vi "Search for Target.vi"(0 "Target":T2, 1 "Focus and Tracking":T3, 3 "Calibration":T5, 5 "Tip":T1, 7 "Refocus Step [um]":dbl=2.0, 9 "Max Distance [um]":dbl=50.0, 11 "Error In":errorcluster, 12 "System of Reference Interface":T4, 13 "Z direction":i8(ring)=-1 items=["Positive"=1, "Negative"=-1], 14 "Abort":refnum<vi>) -> (4 "Target Lost":bool, 6 "Scope Error":bool, 15 "Error Out":errorcluster)   [LabVIEW 2012, in "Targeting Unit.lvlib"]
uses:
  Targeting Unit.lvlib
  <vilib>/Analysis/Matrix/Datatypes/RealMatrix.ctl
  <vilib>/Analysis/NI_AALBase.lvlib
  <vilib>/Analysis/Matrix/NI_Matrix.lvlib
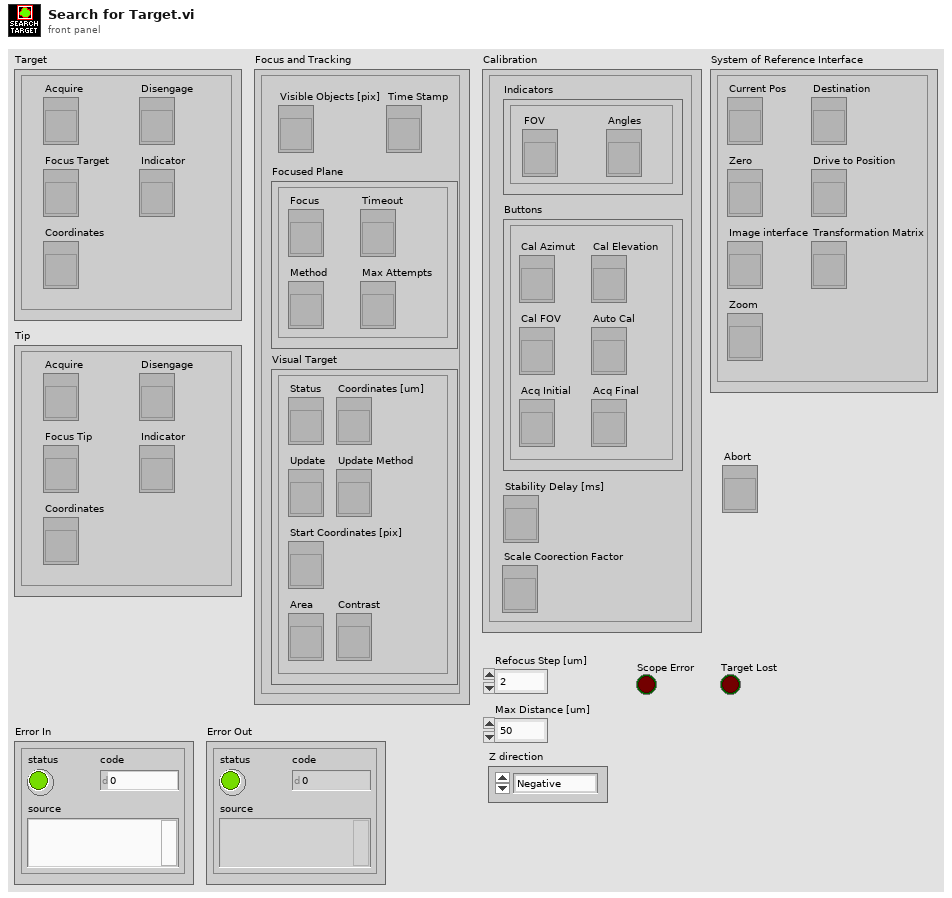
[diagram p1: front panel]
types:
  T1 = cluster{"Coordinates":refnum<vi>, "Acquire":refnum<vi>, "Disengage":refnum<vi>, "Indicator":refnum<vi>, "Focus Tip":refnum<vi>}
  T2 = cluster{"Coordinates":refnum<vi>, "Acquire":refnum<vi>, "Disengage":refnum<vi>, "Indicator":refnum<vi>, "Focus Target":refnum<vi>}
  T3 = cluster{"Focused Plane":cluster{"Focus":refnum<vi>, "Timeout":refnum<vi>, "Max Attempts":refnum<vi>, "Method":refnum<vi>}, "Time Stamp":refnum<vi>, "Visual Target":cluster{"Coordinates [um]":refnum<vi>, "Status":refnum<vi>, "Update":refnum<vi>, "Update Method":refnum<vi>, "Start Coordinates [pix]":refnum<vi>, "Area":refnum<vi>, "Contrast":refnum<vi>}, "Visible Objects [pix]":refnum<vi>}
  T4 = cluster{"Current Pos":refnum<vi>, "Image interface":refnum<vi>, "Transformation Matrix":refnum<vi>, "Zero":refnum<vi>, "Destination":refnum<vi>, "Drive to Position":refnum<vi>, "Zoom":refnum<vi>}
  T5 = cluster{"Indicators":cluster{"FOV":refnum<vi>, "Angles":refnum<vi>}, "Buttons":cluster{"Cal FOV":refnum<vi>, "Cal Azimut":refnum<vi>, "Cal Elevation":refnum<vi>, "Auto Cal":refnum<vi>, "Acq Initial":refnum<vi>, "Acq Final":refnum<vi>}, "Stability Delay [ms]":refnum<vi>, "Scale Coorection Factor":refnum<vi>}
  T6 = cluster{"X [um]":dbl, "Y [um]":dbl, "Z [um]":dbl}
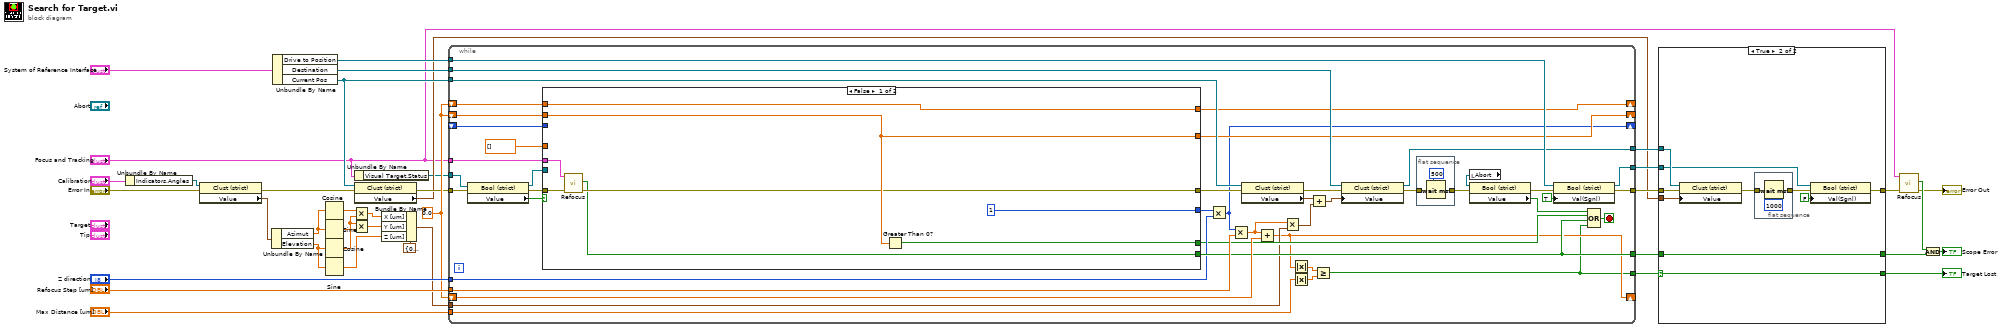
[diagram p0: block diagram]
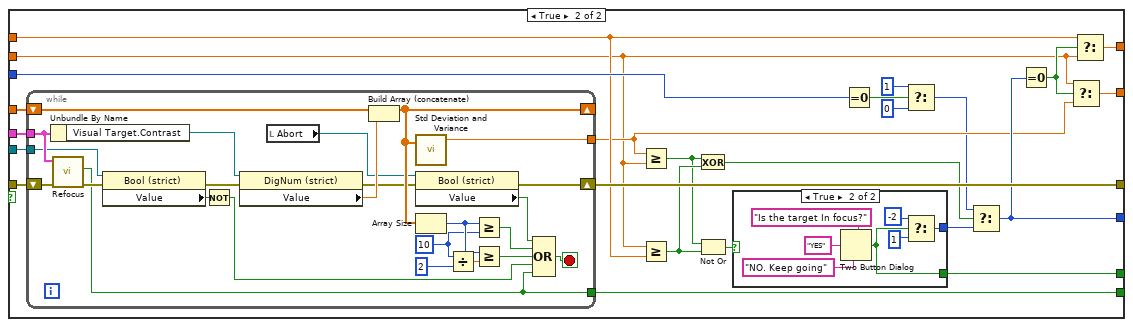
[diagram p3: hidden frame]
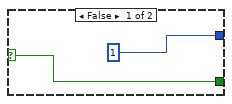
[diagram p4: hidden frame]
diagram:
  w32 = 0.0 ("Value")
  n1 = Unbundle By Name("Calibration") -> ("Indicators.Angles"=w24:refnum<vi>)
  n2 = property class="Clust (strict)"(reference=w24, error in="Error In") -> (error out=w23:errorcluster, "Value"=w28:cluster{"Azimut":dbl, "Elevation":dbl})  [unwired: 1 out]
  n3 = Unbundle By Name(w28) -> ("Azimut"=w30:dbl, "Elevation"=w25:dbl)
  n4 = Unbundle By Name("System of Reference Interface") -> ("Drive to Position"=w18:refnum<vi>, "Destination"=w16:refnum<vi>, "Current Pos"=w17:refnum<vi>)
  n5 = Cosine(x=w30) -> (cos(x)=w1:dbl)
  n6 = Sine(x=w30) -> (sin(x)=w2:dbl)
  n7 = Cosine(x=w25) -> (cos(x)=w27:dbl)
  n8 = Sine(x=w25) -> (sin(x)=w29:dbl)
  n9 = Multiply(x=w1, y=w27) -> (x*y=w11:dbl)
  n10 = Multiply(x=w27, y=w2) -> (x*y=w12:dbl)
  n11 = Unbundle By Name("Focus and Tracking") -> ("Visual Target.Status"=w10:refnum<vi>)
  n12 = property class="Clust (strict)"(reference=w17, error in=w23) -> (error out=w22:errorcluster, "Value"=w15:T6)  [unwired: 1 out]
  n13 = Bundle By Name(cluster=T6 {"X [um]"=0.0, "Y [um]"=0.0, "Z [um]"=0.0} ("y"), "X [um]"=w11, "Y [um]"=w12, "Z [um]"=w29) -> (w9:T6)
  n14 = while {
    tunnel: "Refocus Step [um]" -> [w69]
    tunnel: w22 -> [w60]
    tunnel: "Focus and Tracking" -> [w62]
    tunnel: [w58] -> w21
    shift-right: [w40] -> _
    shift-left: w32 -> [w77]
    tunnel: "Max Distance [um]" -> [w72]
    tunnel: w17 -> [w76]
    tunnel: w18 -> [w75]
    tunnel: [w74] -> w20
    tunnel: [w73] -> w19
    tunnel: "Z direction" -> [w51]
    shift-right: [w61] -> _
    shift-left: w32 -> [w56]
    tunnel: [w39] -> w13
    tunnel: w16 -> [w67]
    tunnel: w9 -> [w42]
    shift-right: [w54] -> _
    shift-left: w32 -> [w55]
    shift-right: [w46] -> _
    shift-left: _ -> [w53]
    tunnel: [w59] -> w14
    tunnel: w10 -> [w44]
    stop <- w68 stop-if-true
    n15 = property class="Bool (strict)"(reference=w44, error in=w60) -> (reference out=w64:refnum<vi>, error out=w63:errorcluster, "Value"=w65:bool)
    n16 = case shown="False" w65 {
      tunnel: w62 -> [w89 w114]
      tunnel: [w86 w99] -> w59
      tunnel: w63 -> [w88 w113]
      tunnel: w64 -> [_ w112]
      tunnel: w56 -> [w90 w95]
      tunnel: [w90 w94] -> w61
      tunnel: [w84 w100] -> w45
      tunnel: [w87 w111] -> w57
      tunnel: dbl[] [] -> [_ w110]
      tunnel: w55 -> [w85 w97]
      tunnel: [w85 w93] -> w54
      tunnel: [i8 1 w108] -> w50
      tunnel: w53 -> [_ w102]
      frame False {
        n17 = call "Refocus.vi"("Error In"=w88, "Focus and Tracking"=w89) -> ("Error Out"=w87:errorcluster, "Error"=w86:bool)  [unwired: 8 in]
        n18 = Greater Than 0?(x=w90) -> (x > 0?=w84:bool)
      }
      frame True {
        n19 = while {
          shift-right: [w126] -> w111
          shift-left: w113 -> [w146]
          tunnel: w114 -> [w144]
          tunnel: [w129] -> w99
          shift-right: [w139] -> _
          shift-left: w110 -> [w140]
          tunnel: [w138] -> w96
          tunnel: w112 -> [w136]
          stop <- w137 stop-if-true
          w131 = 10 ("y")
          n20 = Unbundle By Name(w144) -> ("Visual Target.Contrast"=w142:refnum<vi>)
          n21 = call "Refocus.vi"("Error In"=w146, "Focus and Tracking"=w144) -> ("Error Out"=w147:errorcluster, "Error"=w129:bool)  [unwired: 8 in]
          n22 = property class="Bool (strict)"(reference=w136, error in=w147) -> (error out=w145:errorcluster, "Value"=w143:bool)  [unwired: 1 out]
          n23 = Not(x=w143) -> (.not. x?=w130:bool)
          n24 = property class="DigNum (strict)"(reference=w142, error in=w145) -> (error out=w127:errorcluster, "Value"=w141:dbl)  [unwired: 1 out]
          n25 = local read "Abort"() -> (w124:refnum<vi>)
          n26 = Build Array (concatenate)(w140, w141) -> (w139:dbl[])
          n27 = call <vilib>:"Std Deviation and Variance.vi"("X"=w139) -> ("mean"=w138:dbl)  [unwired: 1 in, 2 out]
          n28 = property class="Bool (strict)"(reference=w124, error in=w127) -> (error out=w126:errorcluster, "Value"=w125:bool)  [unwired: 1 out]
          n29 = Array Size(array=w139) -> (size(s)=w134:i32)
          n30 = Divide(x=w131, y=2) -> (x/y=w132:dbl)
          n31 = Greater Or Equal?(x=w134, y=w131) -> (x >= y?=w135:bool)
          n32 = Greater Or Equal?(x=w134, y=w132) -> (x >= y?=w128:bool)
          n33 = Compound Arithmetic op=OR(w125, w135, w128, w130, w129) -> (w137:bool)
        }
        n34 = Greater Or Equal?(x=w96, y=w95) -> (x >= y?=w106:bool)
        n35 = Greater Or Equal?(x=w95, y=w97) -> (x >= y?=w109:bool)
        n36 = Exclusive Or(1:w109, 2:w106) -> (0:w107:bool)
        n37 = Not Or(1:w109, 2:w106) -> (0:w101:bool)
        n38 = case shown="True" w101 {
          selector: w101 -> [w116 _]
          tunnel: [w116 w118] -> w100
          tunnel: [i8 1 ("f") w117] -> w91
          frame False {
          }
          frame True {
            n39 = Two Button Dialog(message="Is the target In focus?", 1:"NO. Keep going" ("F button name (\"Cancel\")"), 2:"YES" ("T button name (\"OK\")")) -> (T button?=w118:bool)
            n40 = Select(t=i8 -2 ("f"), s=w118, f=i8 1) -> (s? t:f=w117:i8)
          }
        }
        n41 = Equal To 0?(x=w102) -> (x = 0?=w105:bool)
        n42 = Select(t=i8 1 ("f"), s=w105, f=i8 0) -> (s? t:f=w92:i8)
        n43 = Select(t=w92, s=w107, f=w91) -> (s? t:f=w108:i8)
        n44 = Equal To 0?(x=w108) -> (x = 0?=w98:bool)
        n45 = Select(t=w95, s=w98, f=w96) -> (s? t:f=w94:dbl)
        n46 = Select(t=w97, s=w98, f=w95) -> (s? t:f=w93:dbl)
      }
    }
    n47 = Multiply(x=w50, y=w51) -> (x*y=w46:i8)
    n48 = Multiply(x=w46, y=w69) -> (x*y=w43:dbl)
    n49 = property class="Clust (strict)"(reference=w76, error in=w57) -> (error out=w81:errorcluster, "Value"=w80:T6)  [unwired: 1 out]
    n50 = Add(x=w43, y=w77) -> (x+y=w40:dbl)
    n51 = Multiply(x=w43, y=w42) -> (x*y=w66:T6)
    n52 = Absolute Value(x=w40) -> (abs(x)=w70:dbl)
    n53 = Absolute Value(x=w72) -> (abs(x)=w71:dbl)
    n54 = Add(x=w80, y=w66) -> (x+y=w79:T6)
    n55 = Greater Or Equal?(x=w70, y=w71) -> (x >= y?=w39:bool)
    n56 = property class="Clust (strict)"(reference=w67, error in=w81, "Value"=w79) -> (reference out=w74:refnum<vi>, error out=w78:errorcluster)
    n57 = flat-sequence {
      tunnel: [w149] -> w49
      tunnel: w78 -> [w149]
      frame #0 {
        n58 = Wait (ms)(milliseconds to wait=u32 500) -> ()  [unwired: 1 out]
      }
    }
    n59 = local read "Abort"() -> (w41:refnum<vi>)
    n60 = property class="Bool (strict)"(reference=w41, error in=w49) -> (error out=w48:errorcluster, "Value"=w47:bool)  [unwired: 1 out]
    n61 = property class="Bool (strict)"(reference=w75, error in=w48, "Val(Sgnl)"=TRUE ("Value")) -> (reference out=w73:refnum<vi>, error out=w58:errorcluster)
    n62 = Compound Arithmetic op=OR(w47, w45, w59, w39) -> (w68:bool)
  }
  n63 = case shown="True" w13 {
    selector: w13 -> [w150 w155]
    tunnel: w21 -> [w152 w162]
    tunnel: w15 -> [_ w161]
    tunnel: w20 -> [_ w160]
    tunnel: w19 -> [_ w159]
    tunnel: [w152 w154] -> w8
    tunnel: w14 -> [w151 w153]
    tunnel: [w151 w153] -> w5
    tunnel: [w150 w155] -> w34
    frame False {
    }
    frame True {
      n64 = property class="Clust (strict)"(reference=w160, error in=w162, "Value"=w161) -> (error out=w157:errorcluster)  [unwired: 1 out]
      n65 = flat-sequence {
        tunnel: [w164] -> w156
        tunnel: w157 -> [w164]
        frame #0 {
          n66 = Wait (ms)(milliseconds to wait=u32 1000) -> ()  [unwired: 1 out]
        }
      }
      n67 = property class="Bool (strict)"(reference=w159, error in=w156, "Val(Sgnl)"=FALSE ("Value")) -> (error out=w154:errorcluster)  [unwired: 1 out]
    }
  }
  "Target Lost" <- w34
  n68 = call "Refocus.vi"("Error In"=w8, "Focus and Tracking"="Focus and Tracking") -> ("Error Out"=→"Error Out":errorcluster, "Error"=w6:bool)  [unwired: 8 in]
  n69 = And(x=w6, y=w5) -> (x .and. y?=→"Scope Error":bool)
